vi "FileBLFOpen_1.vi"() -> ()   [LabVIEW 2015]
doc: "This is a demo VI to show how the Read Write BLF API works.\n\n-------------\nBrian Hoover (Hooovahh)"
uses:
  BLF/Controls/Cluster - CAN Frame.ctl
  BLF/Controls/Enum - CAN Data Type.ctl
  BLF/Read Write BLF.lvclass/Read Write BLF.ctl
  GetBinlogdllpath.vi
  <vilib>/Utility/file.llb/Application Directory.vi
  <vilib>/Utility/libraryn.llb/Check if File or Folder Exists.vi
  <vilib>/Utility/error.llb/Error Cluster From Error Code.vi
  <vilib>/regexp/Match Regular Expression.xnode
  BLF/Read Write BLF.lvclass
panel:
  out "error out 4":errorcluster
  out "error out 3":errorcluster
  out "error out 2":errorcluster
  out "子匹配 4":string
  out "子匹配 3":string
  out "子匹配 2":string
  out "子匹配 1":string
  out "日期/时间字符串":string
  out "时间字符串":string
  out "日期字符串":string
  out "基时间秒":dbl format="%#_6f"
  out "timestamp":timestamp
  out "payload":u8[](array[numeric])
  out "identifier":u32
  in  "file path (dialog if empty)":path caption="文件路径 （空时为对话框）"
  out "Object Count":u32
  out "error out":errorcluster
  out "Read Frames":T1[](array[typedef]) {"type" items=["CAN Data"=0, "CAN Remote"=1, "CAN Bus Error"=2, "CAN 2.0 Data"=8, "CAN FD Data"=16, "CAN FD+BRS Data"=24, "J1939 Data"=192, "Delay"=224, "Log Trigger"=225, "Start Trigger"=226]; "payload" format="%x"; "timestamp" format="%<%.7X\n%x>T"; "identifier" format="%x"}
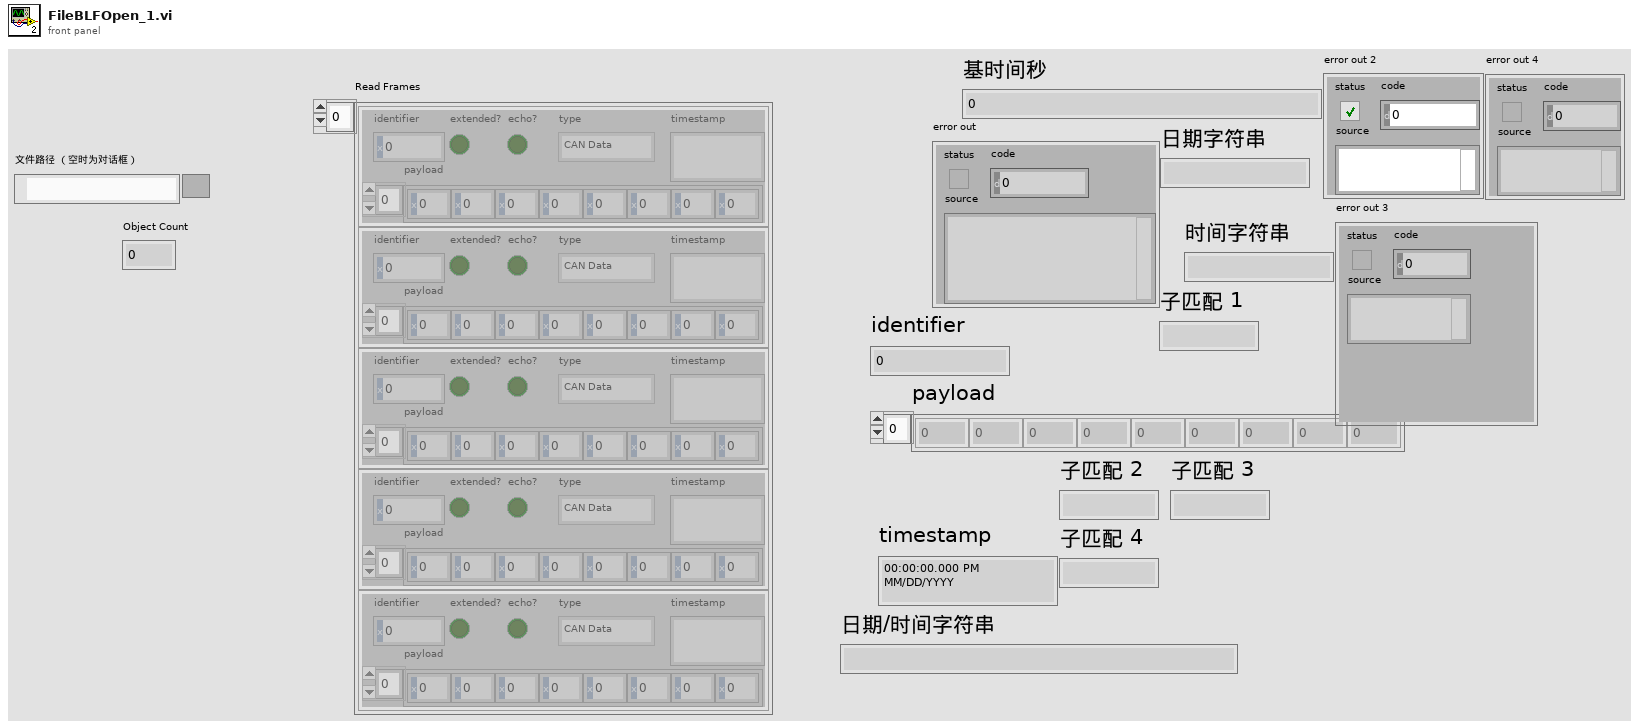
[diagram p1: front panel]
types:
  T1 = typedef "Read Write BLF.lvclass/Cluster - CAN Frame.ctl" = cluster{"timestamp":timestamp, "payload":u8[], "identifier":u32, "extended?":bool, "echo?":bool, "type":T2}
  T2 = typedef "Read Write BLF.lvclass/Enum - CAN Data Type.ctl" = u8
  T3 = cluster{"基时间字符串":string, "基时间秒":dbl, "基时间标识":timestamp}
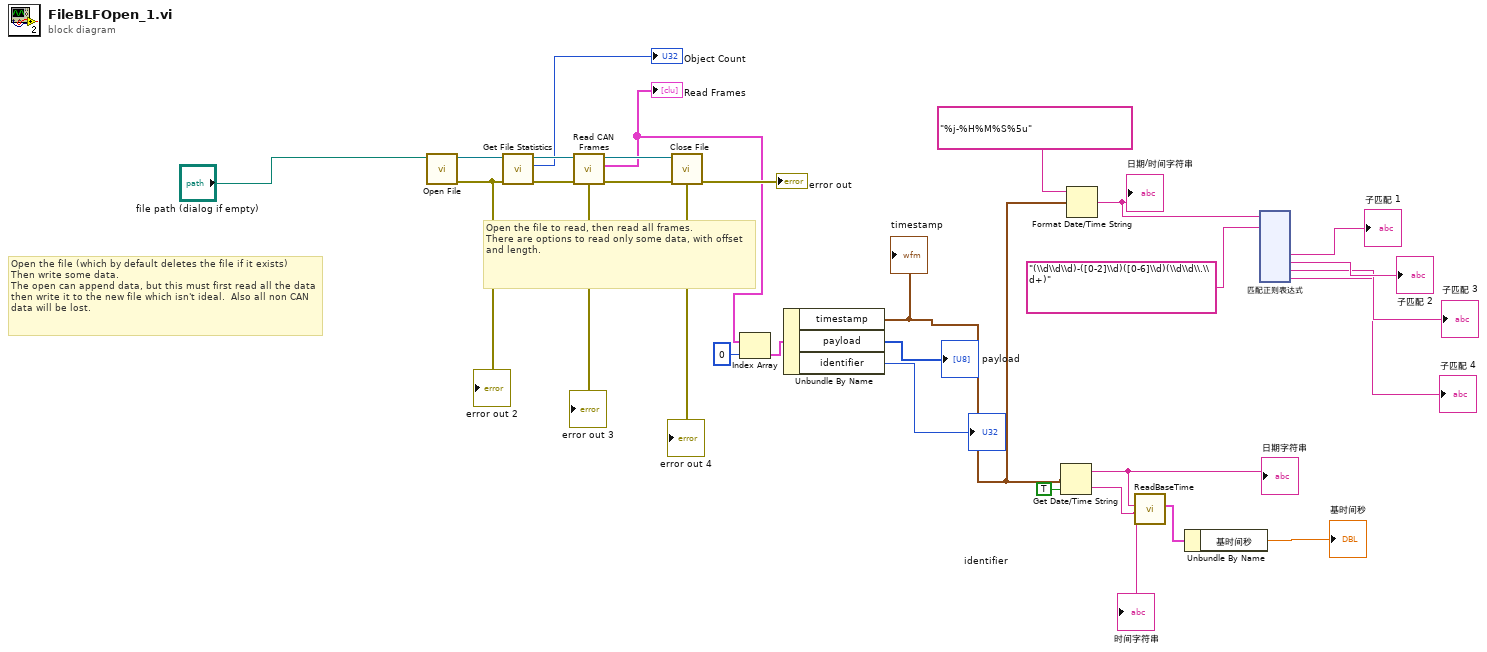
[diagram p0: block diagram]
diagram:
  # "Open the file to read, then read all frames.\nThere are options to read only some data, with offset and length."
  # "Open the file (which by default deletes the file if it exists)\nThen write some data.\nThe open can append data, but this must first read all the data then write it to the new file which isn't ideal.  Also all non CAN data will be lost."
  n1 = call "Open File.vi"("Log Path"="file path (dialog if empty)") -> ("error out"=w25:errorcluster, "BLF File"=w22:refnum<class "Read Write BLF.lvclass">)  [unwired: 9 in]
  "error out 2" <- w25
  n2 = call "Get File Statistics.vi"("error in (no error)"=w25, "Read Write BLF in"=w22) -> ("error out"=w23:errorcluster, "Object Count"=→"Object Count":u32, "Read Write BLF out"=w21:refnum<class "Read Write BLF.lvclass">)  [unwired: 3 in, 4 out]
  "error out 3" <- w23
  n3 = call "Read CAN Frames.vi"("error in (no error)"=w23, "BLF File In"=w21) -> ("error out"=w27:errorcluster, "CAN Frames"=w18:T1[], "BLF File Out"=w26:refnum<class "Read Write BLF.lvclass">)  [unwired: 6 in, 1 out]
  "Read Frames" <- w18
  "error out 4" <- w27
  n4 = call "Close File.vi"("error in (no error)"=w27, "BLF File"=w26) -> ("error out"=→"error out":errorcluster)  [unwired: 8 in, 1 out]
  n5 = Index Array(array=w18, index=0 ("索引")) -> (element=w16:T1)
  n6 = Unbundle By Name(w16) -> ("timestamp"=w8:timestamp, "payload"=→"payload":u8[], "identifier"=→"identifier":u32)
  "timestamp" <- w8
  n7 = Get Date/Time String(seconds (now)=w8, want seconds? (F)=TRUE ("需要秒？(F)")) -> (date string=w12:string, time string=w11:string)  [unwired: 1 in]
  "日期字符串" <- w12
  "时间字符串" <- w11
  n8 = Format Date/Time String(time format string (%c)="%j-%H%M%S%5u" ("时间格式字符串(%c)"), seconds (now)=w8) -> (date/time string=w6:string)  [unwired: 1 in]
  "日期/时间字符串" <- w6
  n9 = call "ReadBaseTime.vi"("时间字符"=w11, "日期字符"=w12) -> ("基时间簇"=w10:T3)  [unwired: 7 in]
  n10 = Unbundle By Name(w10) -> ("基时间秒"=→"基时间秒":dbl)
  n11 = xnode "匹配正则表达式"("输入字符串"=w6, "正则表达式"="(\\d\\d\\d)-([0-2]\\d)([0-6]\\d)(\\d\\d\\.\\d+)") -> ("子匹配 1"=→"子匹配 1":string, "子匹配 2"=→"子匹配 2":string, "子匹配 3"=→"子匹配 3":string, "子匹配 4"=→"子匹配 4":string)  [unwired: 4 in, 5 out]
